vi "ALTS Delete User Information v1.0.vi"(8 "error in (no error)":errorcluster, 10 "Add(T)/Edit(F)":bool=TRUE, 11 "User Name":string) -> (0 "error out":errorcluster, 3 "Deleted?":bool)   [LabVIEW 2013]
doc: "This VI is used to delete the user information completely from the registry. The output of this VI describes whether the user information is deleted or not."
uses:
  <vilib>/Utility/config.llb/NI_LVConfig.lvlib
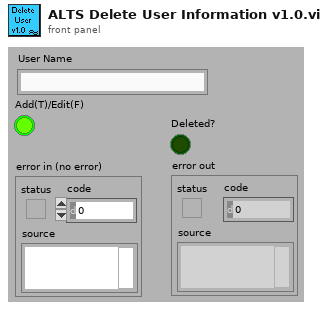
[diagram p1: front panel]
types:
  T1 = typedef "NI_LVConfig.lvlib/Config Data RefNum.ctl" = refnum<k1>
  T2 = enum16{"OK", "CANCEL", "ABORT", "RETRY", "IGNORE", "YES", "NO"}
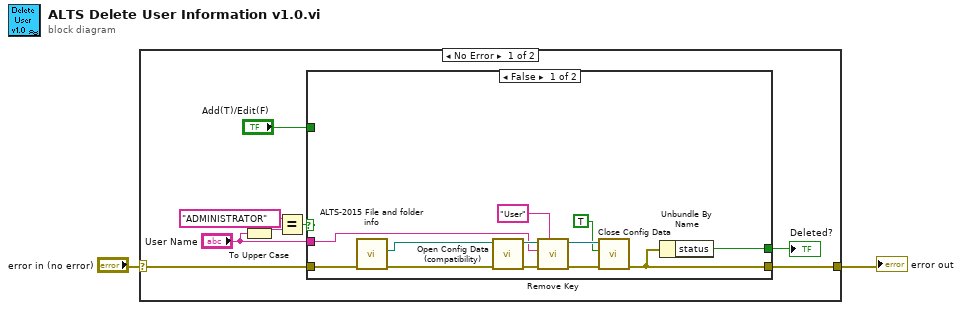
[diagram p0: block diagram]
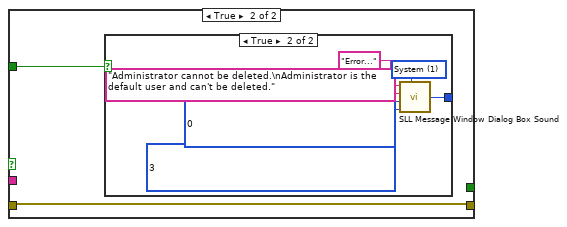
[diagram p2: hidden frame]
diagram:
  n1 = case shown="No Error" "error in (no error)" {
    selector: "error in (no error)" -> [w10 w31]
    tunnel: [w9 w31] -> w1
    frame No Error {
      n2 = To Upper Case(1:"User Name") -> (0:w4:string)
      n3 = Equal?(x="ADMINISTRATOR", y=w4) -> (x = y?=w8:bool)
      n4 = case shown="False" w8 {
        tunnel: w10 -> [w12 w24]
        tunnel: [w15 w24] -> w9
        tunnel: "User Name" -> [w19 _]
        tunnel: "Add(T)/Edit(F)" -> [_ w23]
        tunnel: [w14 _] -> w5
        frame False {
          n5 = call "ALTS-2015 File and folder info.vi"("error in (no error)"=w12) -> ("error out"=w13:errorcluster, "INI file path"=w11:path)  [unwired: 2 in, 7 out]
          n6 = call <vilib>:"Open Config Data (compatibility).vi"("error in (no error)"=w13, "configuration file path"=w11) -> ("error out"=w22:errorcluster, "refnum"=w21:T1)  [unwired: 7 in, 1 out]
          n7 = call <vilib>:"Remove Key.vi"("section"="User", "error in (no error)"=w22, "key"=w19, "refnum"=w21) -> ("error out"=w18:errorcluster, "refnum out"=w17:T1)  [unwired: 5 in, 1 out]
          n8 = call <vilib>:"Close Config Data.vi"("error in (no error)"=w18, "write file if changed (T)"=TRUE ("write configuration file? (F)"), "refnum"=w17) -> ("error out"=w15:errorcluster)  [unwired: 7 in, 1 out]
          n9 = Unbundle By Name(w15) -> ("status"=w14:bool)
        }
        frame True {
          n10 = case shown="True" w23 {
            tunnel: [_ w30] -> _
            frame False {
            }
            frame True {
              w25 = 1 items=["Application", "System", "Task"] ("modality (0)")
              n11 = call <userlib>:"SLL Message Window Dialog Box Sound.vi"("Modality (0)"=w25, "Icon (0:None)"=3 ("icon (0:None)"), "Buttons (0:OK)"=0 ("buttons (0:OK)"), "Message (\"\")"="Administrator cannot be deleted.\nAdministrator is the default user and can't be deleted.", "Window Title (\"\")"="Error...") -> ("Button Pressed"=w30:T2)  [unwired: 1 in]
            }
          }
        }
      }
      "Deleted?" <- w5
    }
    frame Error {
    }
  }
  "error out" <- w1
